vi "Toolbar Initialise.vi"(3 "Container State":T4, 4 "Previous State":variant=variant(cluster{"Buttons Displayed":i32, "Button States":cluster{"Off Picture":picture, "On Picture":picture, "Hover  Picture":picture, "Type":enum16{"Transitory", "Latching"}, "State":enum16{"Off", "Hover", "On", "Disabled"}}[]} {"Buttons Displayed"=3, "Button States"=[{"Off Picture"=bytes[1758], "On Picture"=bytes[1758], "Hover  Picture"=bytes[1758], "Type"=enum."Transitory", "State"=enum."Off"}, {"Off Picture"=bytes[1758], "On Picture"=bytes[1758], "Hover  Picture"=bytes[1758], "Type"=enum."Transitory", "State"=enum."Off"}, {"Off Picture"=bytes[1758], "On Picture"=bytes[1758], "Hover  Picture"=bytes[1758], "Type"=enum."Transitory", "State"=enum."Off"}]}), 5 "Previous Version":T3={"Major"=1, "Minor"=0, "Fix"=0, "Build"=0}) -> (2 "Current State":T1={"Buttons Displayed"=0, "Button States"=[], "Button Size"=0, "Button Style"=enum."Classic", "Active Button"=0, "Force Regen?"=FALSE, "Tip String Ref"=refnum})   [LabVIEW 2012, in "Toolbar.xctl"]
doc: "Standard XControl Initialise ability"
uses:
  Toolbar.xctl
  Toolbar State.ctl
  Button_Class/Button.lvclass
  Button_Class/Type Defs/Button Style.ctl
  <vilib>/_xctls/Container State.ctl
  <vilib>/_xctls/Version.ctl
  <vilib>/_xctls/XControlSupport.lvlib
panel:
  in  "Default Indicator State":T1={"Buttons Displayed"=0, "Button States"=[], "Button Size"=0, "Button Style"=enum."Classic", "Active Button"=0, "Force Regen?"=FALSE, "Tip String Ref"=refnum}
  in  "Default Control State":T1={"Buttons Displayed"=5, "Button States"=[refnum, refnum, refnum, refnum, refnum, refnum], "Button Size"=32, "Button Style"=enum."Classic", "Active Button"=0, "Force Regen?"=FALSE, "Tip String Ref"=refnum}
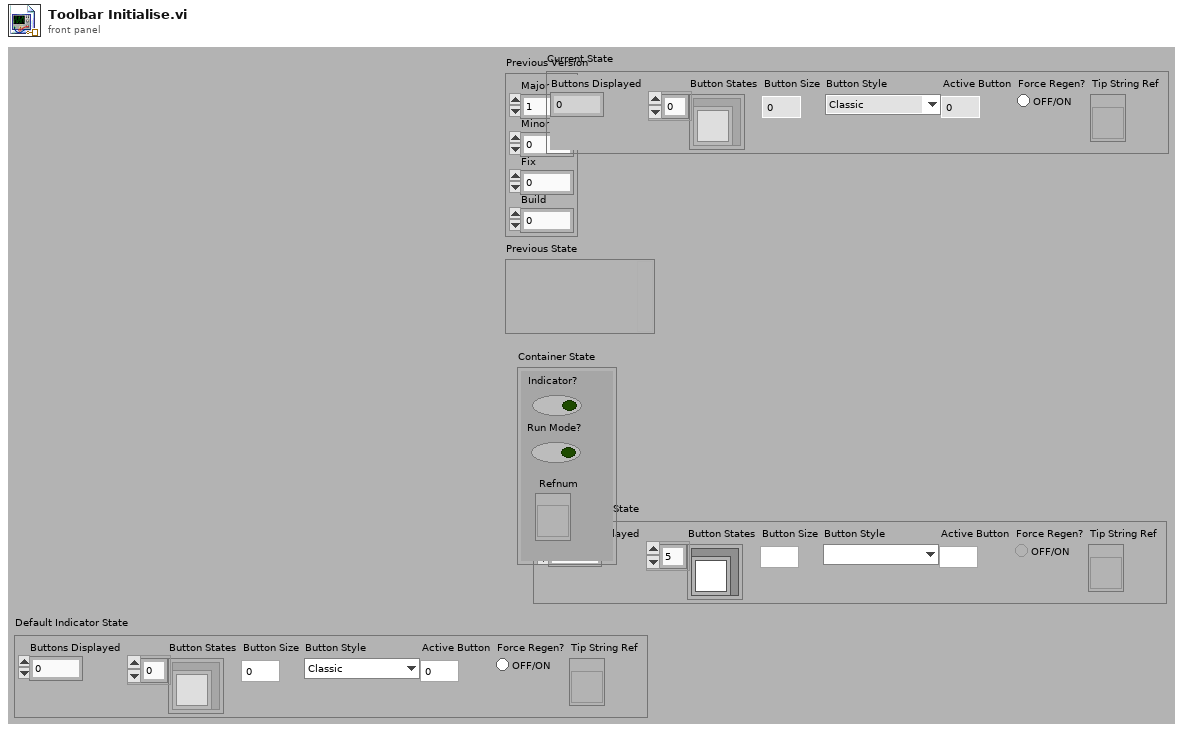
[diagram p1: front panel]
types:
  T1 = typedef "Toolbar.xctl/Toolbar State.ctl" = cluster{"Buttons Displayed":i32, "Button States":refnum<class "Button.lvclass">[], "Button Size":i32, "Button Style":T2, "Active Button":i32, "Force Regen?":bool, "Tip String Ref":refnum<vi>}
  T2 = typedef "Button.lvclass/Button Style.ctl" = enum16{"System", "Modern", "Classic", "Rounded", "Silver", "Ni Theme", "Metallic"}
  T3 = typedef "XControlSupport.lvlib/Version.ctl" = cluster{"Major":u16, "Minor":u16, "Fix":u16, "Build":u16}
  T4 = typedef "XControlSupport.lvlib/Container State.ctl" = cluster{"Indicator?":bool, "Run Mode?":bool, " Refnum":refnum<vi>}
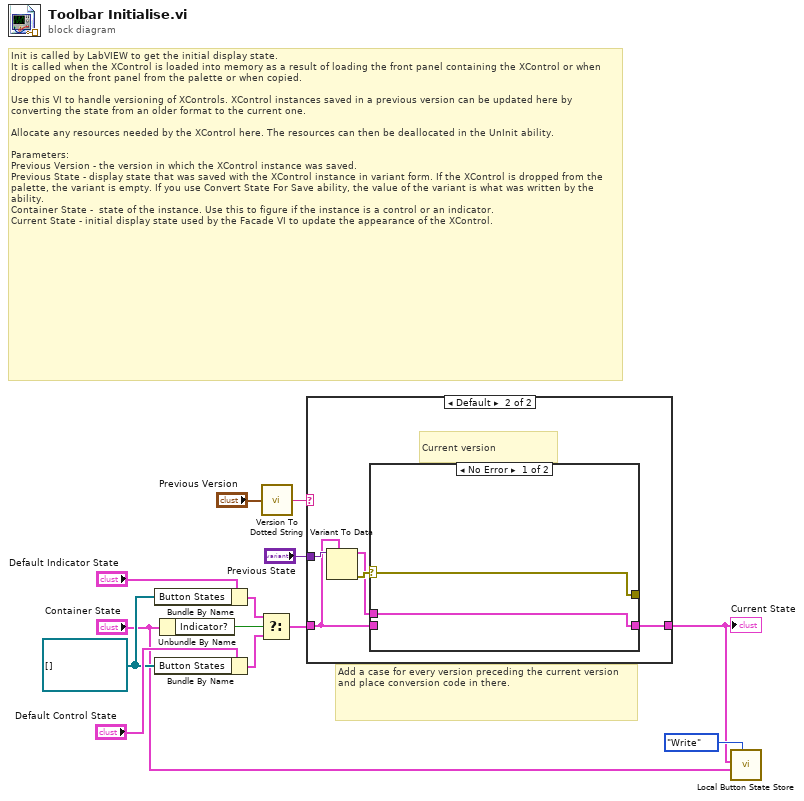
[diagram p0: block diagram]
diagram:
  w4 = refnum<class "Button.lvclass">[] []
  # "Add a case for every version preceding the current version and place conversion code in there."
  # "Init is called by LabVIEW to get the initial display state.\nIt is called when the XControl is loaded into memory as a result of loading the front panel containing the XControl or when dropped on the front panel from the palette or when copied.\n\nUse this VI to handle versioning of XControls. XControl instances saved in a previous version can be updated here by converting the state from an older format to the current one.\n\nAllocate any resources needed by the XControl here. The resources can then be deallocated in the UnInit ability.\n\nParameters:\nPrevious Version - the version in which the XControl instance was saved.\nPrevious State - display state that was saved with the XControl instance in variant form. If the XControl is dropped from the palette, the variant is empty. If you use Convert State For Save ability, the value of the variant is what was written by the ability. \nContainer State -  state of the instance. Use this to figure if the instance is a control or an indicator.\nCurrent State - initial display state used by the Facade VI to update the appearance of the XControl."
  n1 = Bundle By Name(cluster="Default Indicator State", "Button States"=w4) -> (w6:T1)
  n2 = Bundle By Name(cluster="Default Control State", "Button States"=w4) -> (w5:T1)
  n3 = Unbundle By Name("Container State") -> ("Indicator?"=w10:bool)
  n4 = Select(t=w6, s=w10, f=w5) -> (s? t:f=w9:T1)
  n5 = call <vilib>:"Version To Dotted String.vi"("Version"="Previous Version") -> ("String Version"=w7:string)
  n6 = case shown="Default" w7 {
    tunnel: "Previous State" -> [_ w19]
    tunnel: [w14 w15] -> w2
    tunnel: w9 -> [w14 w16]
    frame "0.0.0.0" {
      # "Just created, use default state"
    }
    frame Default {
      # "Current version"
      n7 = Variant To Data(type=w16, Variant=w19) -> (data=w17:T1, error out=w18:errorcluster)  [unwired: 1 in]
      n8 = case shown="No Error" w18 {
        selector: w18 -> [w21 w22]
        tunnel: w17 -> [w20 _]
        tunnel: [w20 w23] -> w15
        tunnel: w16 -> [_ w23]
        tunnel: [w21 w22] -> _
        frame No Error {
        }
        frame Error {
          # "Error converting previously \nsaved state. Use default instead."
        }
      }
    }
  }
  "Current State" <- w2
  n9 = call "Local Button State Store.vi"("Operation"=enum16{"Read", "Write"}."Write", "Container State"="Container State", "Display State In"=w2) -> ()  [unwired: 2 in, 7 out]
